vi "Transition Requested.vi"(11 "statemachine":refnum<class "statemachine.lvclass">) -> (2 "Transition Requested?":bool, 3 "statemachine":refnum<class "statemachine.lvclass">)   [LabVIEW 2020, in "eos.lvlib" / "statemachine.lvclass"]
uses:
  statemachine.lvclass
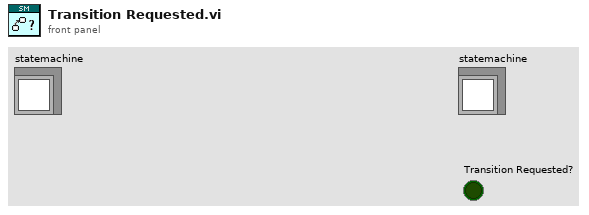
[diagram p1: front panel]
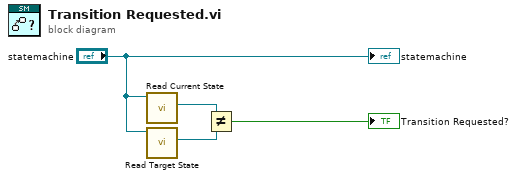
[diagram p0: block diagram]
diagram:
  n1 = call "Read Current State.vi"("statemachine in"="statemachine") -> ("Current State"=w3:refnum<class "state.lvclass">)  [unwired: 9 in, 1 out]
  n2 = call "Read Target State.vi"("statemachine in"="statemachine") -> ("Target State"=w2:refnum<class "state.lvclass">)  [unwired: 9 in, 1 out]
  n3 = Not Equal?(x=w3, y=w2) -> (x != y?=→"Transition Requested?":bool)
  "statemachine" <- "statemachine"
